vi "Sequence Init.vi"(8 "error in (no error)":errorcluster, 11 "MSX-E3701 in":refnum<class "MSX-E3701.lvclass">) -> (0 "error out":errorcluster, 3 "MSX-E3701 out":refnum<class "MSX-E3701.lvclass">)   [LabVIEW 2014, in "MSX-E3701.lvlib" / "MSX-E3701.lvclass"]
doc: "Inicializa el Channel Mask en el programa, según si se lo cargo por el usuario o por sus valores que trae por defecto."
uses:
  MSX-E3701.lvclass
  DriverMasterSync/build/DriverMasterSync.lvlibp/Modules/HAL/DriverMasterSync/DriverMasterSyncClass/DriverMasterSync.lvclass
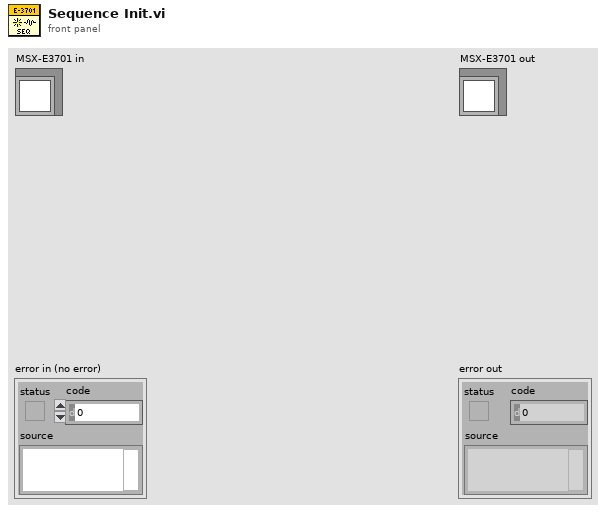
[diagram p1: front panel]
types:
  T1 = typedef "DriverMasterSync.lvlibp/HAL Config Data.ctl" = cluster{"HWSync Index":u32, "Driver Name":string, "Channel Mask":u64}
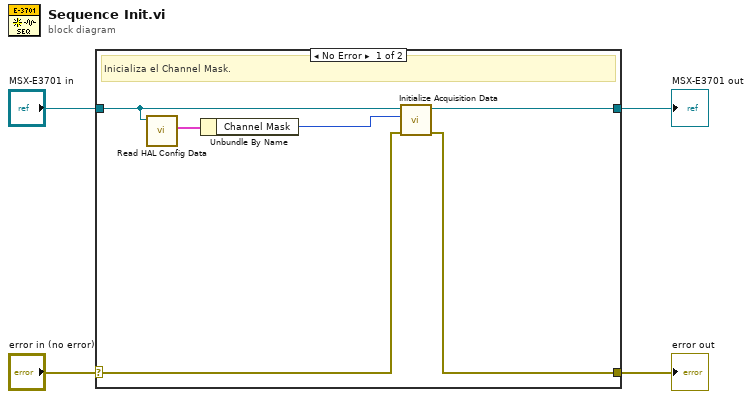
[diagram p0: block diagram]
diagram:
  n1 = case shown="No Error" "error in (no error)" {
    selector: "error in (no error)" -> [w10 w12]
    tunnel: [w9 w12] -> w3
    tunnel: [w5 w11] -> w1
    tunnel: "MSX-E3701 in" -> [w6 w11]
    frame No Error {
      # "Inicializa el Channel Mask."
      n2 = call "Read HAL Config Data.vi"("DriverMasterSync in"=w6) -> ("HAL Config Data"=w7:T1)  [unwired: 8 in, 2 out]
      n3 = Unbundle By Name(w7) -> ("Channel Mask"=w8:u64)
      n4 = call "Initialize Acquisition Data.vi"("error in (no error)"=w10, "Channel Mask"=w8, "DriverMasterSync in"=w6) -> ("error out"=w9:errorcluster, "DriverMasterSync out"=w5:refnum<class "MSX-E3701.lvclass">)  [unwired: 7 in]
    }
    frame Error {
    }
  }
  "error out" <- w3
  "MSX-E3701 out" <- w1
